vi "BusOut.vi"(8 "error in (no error)":errorcluster, 9 "Existing Obj Name":string, 10 "pins":string[](array[string]), 11 "mbed_LVLibrary.lvlib:mbed.lvclass":refnum<class "mbed.lvclass">) -> (0 "error out":errorcluster, 1 "Assigned Name":string, 3 "BusOut.lvclass 2":refnum<class "BusOut.lvclass">)   [LabVIEW 2011, in "mbed_LVLibrary.lvlib" / "BusOut.lvclass"]
uses:
  BusOut.lvclass
  Transport Mechanisms/mbed/mbed.lvclass
  BusOut.lvclass/BusOut.ctl
  <vilib>/regexp/Match Regular Expression.xnode
panel:
  in  "BusOut.lvclass":refnum<class "BusOut.lvclass">
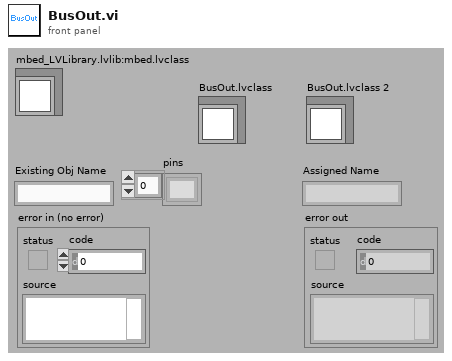
[diagram p1: front panel]
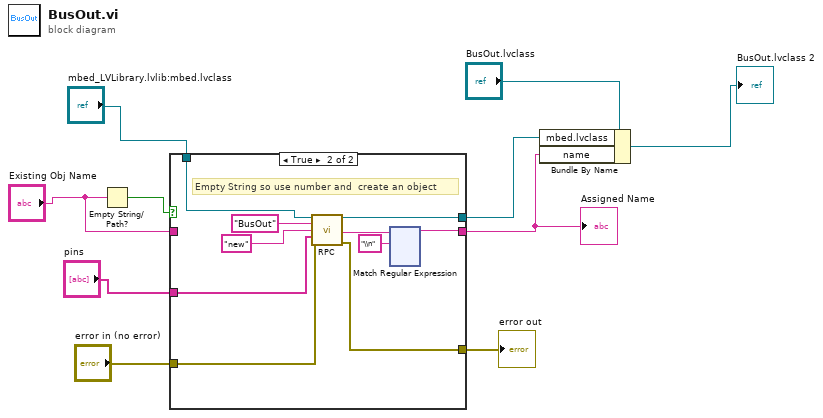
[diagram p0: block diagram]
diagram:
  n1 = Empty String/Path?(string/path="Existing Obj Name") -> (empty?=w8:bool)
  n2 = case shown="True" w8 {
    tunnel: "Existing Obj Name" -> [w13 _]
    tunnel: [w13 w19] -> w7
    tunnel: "mbed_LVLibrary.lvlib:mbed.lvclass" -> [w12 w23]
    tunnel: [w12 w20] -> w9
    tunnel: "pins" -> [_ w16]
    tunnel: "error in (no error)" -> [w11 w15]
    tunnel: [w11 w14] -> w2
    frame False {
      # "String present so just set the class name"
    }
    frame True {
      # "Empty String so use number and  create an object"
      n3 = call-dynamic "RPC.vi"("mbed in"=w23, "Name"="BusOut", "method"="new", "Args"=w16, "error in (no error)"=w15) -> ("mbed out"=w20:refnum<class "mbed.lvclass">, "RPC Result"=w18:string, "error out"=w14:errorcluster)  [unwired: 8 in]
      n4 = xnode "Match Regular Expression"("input string"=w18, "regular expression"="\\n") -> ("before match"=w19:string)  [unwired: 4 in, 4 out]
    }
  }
  "Assigned Name" <- w7
  "error out" <- w2
  n5 = Bundle By Name(cluster="BusOut.lvclass", "mbed.lvclass"=w9, "name"=w7) -> (→"BusOut.lvclass 2":refnum<class "BusOut.lvclass">)
